vi "Export SystemLink State Example.vi"() -> ()   [LabVIEW 2017]
uses:
  SystemLink_States_API.lvlib
panel:
  in  "state destination filepath":path
  out "raw state text":string
  out "state name out":string
  in  "state name":string
  in  "password":string
  in  "username":string
  in  "SystemLink server base URL":string="https://"
  # "SystemLink Server"
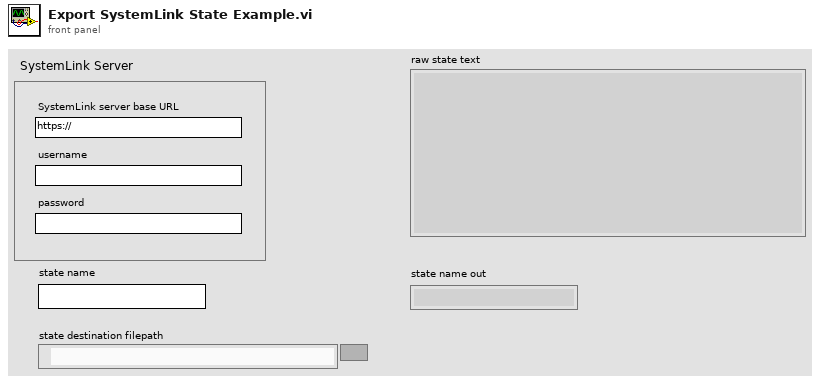
[diagram p1: front panel]
types:
  T1 = typedef "SystemLink_States_API.lvlib/systemlink connection.ctl" = cluster{"client handle out":T2, "SystemLink server base URL":string}
  T2 = typedef "LabVIEWHTTPClient.lvlib/ClientHandle.ctl" = refnum<k1>
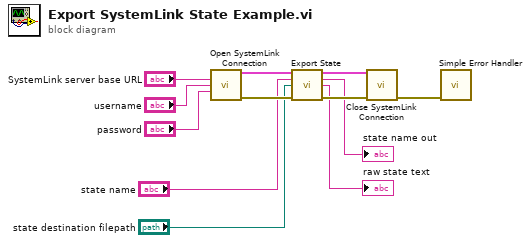
[diagram p0: block diagram]
diagram:
  n1 = call "Open SystemLink Connection.vi"("SystemLink server base URL"="SystemLink server base URL", "username"="username", "password"="password") -> ("SystemLink connection out"=w8:T1, "error out"=w6:errorcluster)  [unwired: 11 in]
  n2 = call "Export State.vi"("SystemLink connection in"=w8, "state name"="state name", "state destination filepath"="state destination filepath", "error in (no error)"=w6) -> ("SystemLink connection out"=w7:T1, "state name out"=→"state name out":string, "raw state text"=→"raw state text":string, "error out"=w5:errorcluster)  [unwired: 8 in]
  n3 = call "Close SystemLink Connection.vi"("SystemLink connection in"=w7, "error in (no error)"=w5) -> ("error out"=w9:errorcluster)  [unwired: 13 in]
  n4 = call <vilib>:"Simple Error Handler.vi"("error in (no error)"=w9) -> ()  [unwired: 4 in, 5 out]
